vi "From U16.vi"(10 "Array":u16[](array[numeric]), 11 "DataType":T1) -> (3 "Numeric":dbl)   [LabVIEW 2021, in "Modbus Master Engine.lvlib"]
uses:
  Modbus Master Engine.lvlib
  Shared/Controls/Data Model/DataType.ctl
  Shared/Modbus Master Shared.lvlib
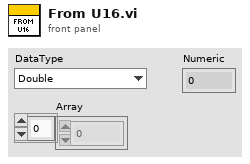
[diagram p1: front panel]
types:
  T1 = typedef "Modbus Master Shared.lvlib/DataType.ctl" = enum16{"Double", "Single", "I64", "I32", "I16", "I8", "U64", "U32", "U16", "U8", "Boolean"}
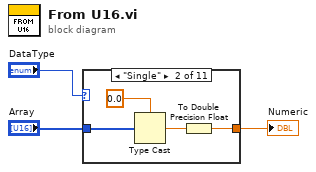
[diagram p0: block diagram]
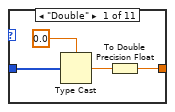
[diagram p2: hidden frame]
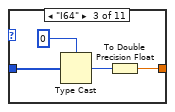
[diagram p3: hidden frame]
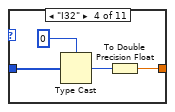
[diagram p4: hidden frame]
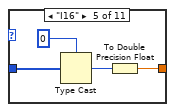
[diagram p5: hidden frame]
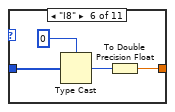
[diagram p6: hidden frame]
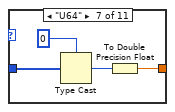
[diagram p7: hidden frame]
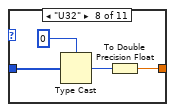
[diagram p8: hidden frame]
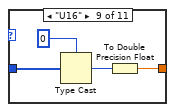
[diagram p9: hidden frame]
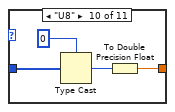
[diagram p10: hidden frame]
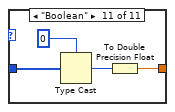
[diagram p11: hidden frame]
diagram:
  n1 = case shown="\"Single\"" "DataType" {
    tunnel: "Array" -> [w5 w10 w14 w18 w22 w26 w30 w34 w38 w42 w46]
    tunnel: [w7 w8 w12 w16 w20 w24 w28 w32 w36 w40 w45] -> w3
    frame "Double" {
      n2 = Type Cast(type=0.0, x=w5) -> (*(type *) &x=w4:dbl)
      n3 = To Double Precision Float(number=w4) -> (double precision float=w7:dbl)
    }
    frame "Single" {
      n4 = Type Cast(type=sgl 0.0, x=w10) -> (*(type *) &x=w9:sgl)
      n5 = To Double Precision Float(number=w9) -> (double precision float=w8:dbl)
    }
    frame "I64" {
      n6 = Type Cast(type=i64 0, x=w14) -> (*(type *) &x=w13:i64)
      n7 = To Double Precision Float(number=w13) -> (double precision float=w12:dbl)
    }
    frame "I32" {
      n8 = Type Cast(type=0, x=w18) -> (*(type *) &x=w17:i32)
      n9 = To Double Precision Float(number=w17) -> (double precision float=w16:dbl)
    }
    frame "I16" {
      n10 = Type Cast(type=i16 0, x=w22) -> (*(type *) &x=w21:i16)
      n11 = To Double Precision Float(number=w21) -> (double precision float=w20:dbl)
    }
    frame "I8" {
      n12 = Type Cast(type=i8 0, x=w26) -> (*(type *) &x=w25:i8)
      n13 = To Double Precision Float(number=w25) -> (double precision float=w24:dbl)
    }
    frame "U64" {
      n14 = Type Cast(type=u64 0, x=w30) -> (*(type *) &x=w29:u64)
      n15 = To Double Precision Float(number=w29) -> (double precision float=w28:dbl)
    }
    frame "U32" {
      n16 = Type Cast(type=u32 0, x=w34) -> (*(type *) &x=w33:u32)
      n17 = To Double Precision Float(number=w33) -> (double precision float=w32:dbl)
    }
    frame "U16" {
      n18 = Type Cast(type=u16 0, x=w38) -> (*(type *) &x=w37:u16)
      n19 = To Double Precision Float(number=w37) -> (double precision float=w36:dbl)
    }
    frame "U8" {
      n20 = Type Cast(type=u8 0, x=w42) -> (*(type *) &x=w41:u8)
      n21 = To Double Precision Float(number=w41) -> (double precision float=w40:dbl)
    }
    frame "Boolean" {
      n22 = Type Cast(type=u8 0, x=w46) -> (*(type *) &x=w44:u8)
      n23 = To Double Precision Float(number=w44) -> (double precision float=w45:dbl)
    }
  }
  "Numeric" <- w3
